vi "Display Unicode Strings in Cluster.vi"() -> ()   [LabVIEW 2009]
panel:
  in  "ASCII":string
  out "Cluster":cluster{"Numeric":dbl, "String":string}
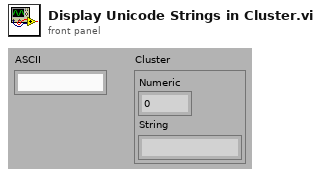
[diagram p1: front panel]
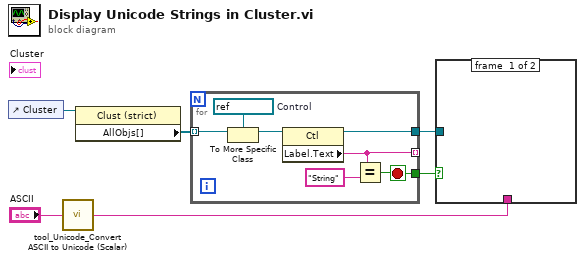
[diagram p0: block diagram]
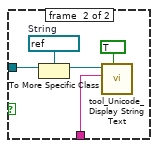
[diagram p2: hidden frame]
diagram:
  n1 = control-ref of="Cluster"() -> (w5:refnum<vi>)
  n2 = call "tool_Unicode_Convert ASCII to Unicode (Scalar).vi"("ASCII"="ASCII") -> ("Unicode"=w1:string)  [unwired: 4 in]
  n3 = property class="Clust (strict)"(reference=w5) -> ("AllObjs[]"=w4:refnum<vi>[])  [unwired: 1 in, 2 out]
  n4 = for {
    tunnel: w4 -> [w12] mode=indexing
    tunnel: [w10] -> _ mode=indexing
    tunnel: [w8] -> w3
    tunnel: [w7] -> w2
    stop <- w8 stop-if-true
    w13 = refnum<vi> refnum  # Control
    n5 = To More Specific Class(target class=w13, reference=w12) -> (specific class reference=w11:refnum<vi>)  [unwired: 1 in, 1 out]
    n6 = property class="Ctl"(reference=w11) -> (reference out=w7:refnum<vi>, "Label.Text"=w10:string)  [unwired: 1 in, 1 out]
    n7 = Equal?(x=w10, y="String") -> (x = y?=w8:bool)
  }
  n8 = case shown="True" w3 {
    tunnel: w2 -> [_ w16]
    tunnel: w1 -> [_ w15]
    frame #0 {
    }
    frame #1 {
      w17 = refnum<vi> refnum  # String
      n9 = To More Specific Class(target class=w17, reference=w16) -> (specific class reference=w18:refnum<vi>)  [unwired: 1 in, 1 out]
      n10 = call "tool_Unicode_Display String Text.vi"("Interpret as Unicode (T)"=TRUE, "String Value"=w15, "String Control Reference"=w18) -> ()  [unwired: 5 in, 2 out]
    }
  }
